vi "Read ID Token.vi"(8 "error in (no error)":errorcluster, 11 "Oauth2 in":refnum<class "Oauth2.lvclass">) -> (0 "error out":errorcluster, 2 "ID Token":T1, 3 "Oauth2 out":refnum<class "Oauth2.lvclass">)   [LabVIEW 2019, in "Oauth2.lvclass"]
doc: "OpenID Connect (OIDC) is an identity layer built on top of the OAuth 2.0 framework. It allows third-party applications to verify the identity of the end-user and to obtain basic user profile information. \n\nOIDC uses JSON web tokens (JWTs), which you can obtain using flows conforming to the OAuth 2.0 specifications.\n\nhttps://auth0.com/docs/secure/tokens/json-web-tokens/json-web-token-structure"
uses:
  Oauth2.lvclass
  OAuthToken/OAuth2 Token Element -- enum.ctl
  Oauth2.lvclass/Oauth2.ctl
  <vilib>/LabVIEW Open Source Project/OpenSerializer.Base64/Base64_ByteLUT.vi
  OAuthToken/OAuthAccessToken.lvclass
  <vilib>/LabVIEW Open Source Project/OpenSerializer.Base64/Serializer.Base64.lvclass
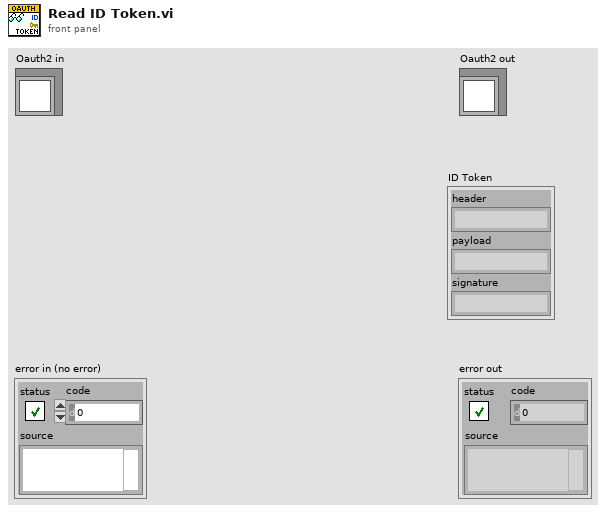
[diagram p1: front panel]
types:
  T1 = cluster{"header":string, "payload":string, "signature":string}
  T2 = typedef "OAuthAccessToken.lvclass/OAuth2 Token Element -- enum.ctl" = enum16{"client_id", "client_secret", "response_type", "scope", "redirect_uri", "error", "error_description", "error_uri", "grant_type", "code", "access_token", "token_type", "expires_in", "username", "password", "refresh_token", "code_challenge", "code_challenge_method", "reverse_proxy_uri", "endpoint element", "prompt", "access_type", "id_token"}
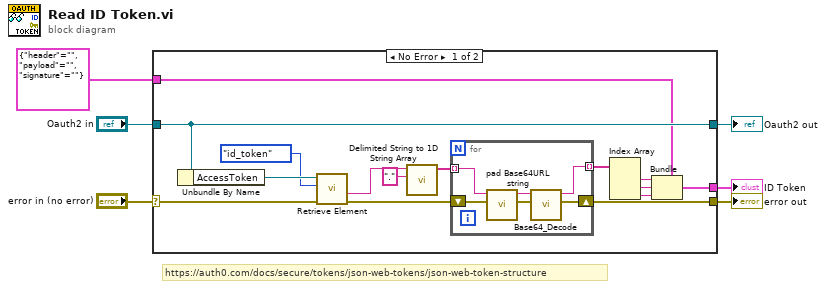
[diagram p0: block diagram]
diagram:
  # "https://auth0.com/docs/secure/tokens/json-web-tokens/json-web-token-structure"
  n1 = case shown="No Error" "error in (no error)" {
    selector: "error in (no error)" -> [w18 w29]
    tunnel: [w16 w29] -> w5
    tunnel: [w21 w30] -> w3
    tunnel: "Oauth2 in" -> [w21 w30]
    tunnel: T1 {"header"="", "payload"="", "signature"=""} -> [w11 w28]
    tunnel: [w7 w28] -> w1
    frame No Error {
      n2 = Unbundle By Name(w21) -> ("AccessToken"=w20:refnum<class "OAuthAccessToken.lvclass">)
      n3 = call "Retrieve Element.vi"("error in (no error)"=w18, "Token element"=OAuth2_Token_Element_--_enum."id_token", "OAuthAccessToken in"=w20) -> ("error out"=w17:errorcluster, "Value"=w14:string)  [unwired: 4 in, 3 out]
      n4 = call <vilib>:"Delimited String to 1D String Array.vi"("delimiter"=".", "delimited string"=w14) -> ("string array"=w13:string[])  [unwired: 9 in]
      n5 = for {
        tunnel: [w27] -> w12 mode=indexing
        shift-right: [w26] -> w16
        shift-left: w17 -> [w25]
        tunnel: w13 -> [w24] mode=indexing
        n6 = call "pad Base64URL string.vi"("error in (no error)"=w25, "Base64URL string"=w24) -> ("error out"=w22:errorcluster, "padded Base64 string"=w23:string)  [unwired: 8 in]
        n7 = call <vilib>:"Base64_Decode.vi"("error in (no error)"=w22, "Base64 String"=w23) -> ("error out"=w26:errorcluster, "Decoded String"=w27:string)  [unwired: 8 in]
      }
      n8 = Index Array(array=w12) -> (element #1=w10:string, element #2=w9:string, element #3=w8:string)  [unwired: 3 in]
      n9 = Bundle(cluster=w11, "header"=w10, "payload"=w9, "signature"=w8) -> (w7:T1)
    }
    frame Error {
    }
  }
  "error out" <- w5
  "Oauth2 out" <- w3
  "ID Token" <- w1
